vi "Convert Array to BMIH.vi"(1 "Array":u8[](array[numeric])) -> (0 "BITMAPINFOHEADER":T1)   [LabVIEW 2013, in "VRI.lvlib"]
uses:
  VRI.lvlib
  _Type Defs/BITMAPINFOHEADER.ctl
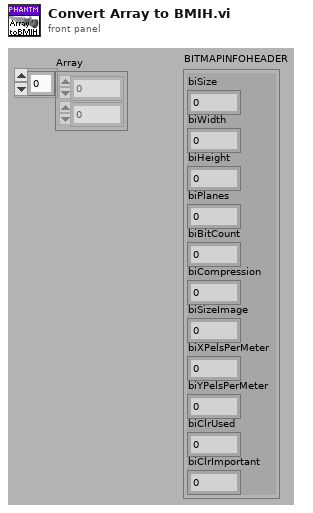
[diagram p1: front panel]
types:
  T1 = typedef "VRI.lvlib/BITMAPINFOHEADER.ctl" = cluster{"biSize":u32, "biWidth":i32, "biHeight":i32, "biPlanes":u16, "biBitCount":u16, "biCompression":u32, "biSizeImage":u32, "biXPelsPerMeter":i32, "biYPelsPerMeter":i32, "biClrUsed":u32, "biClrImportant":u32}
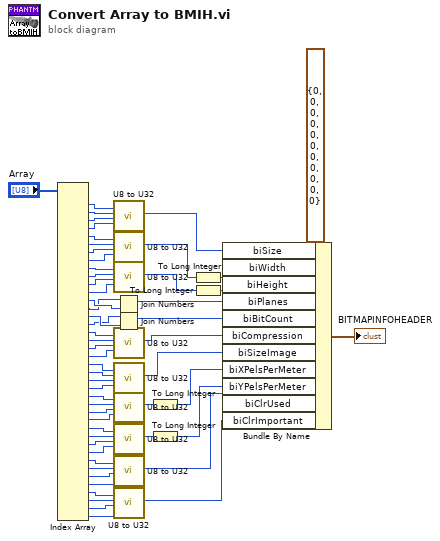
[diagram p0: block diagram]
diagram:
  n1 = Index Array(array="Array") -> (element #1=w7:u8, element #2=w4:u8, element #3=w6:u8, element #4=w5:u8, element #5=w9:u8, element #6=w10:u8, element #7=w11:u8, element #8=w12:u8, element #9=w13:u8, element #10=w14:u8, element #11=w15:u8, element #12=w16:u8, element #13=w56:u8, element #14=w55:u8, element #15=w58:u8, element #16=w57:u8, element #17=w23:u8, element #18=w24:u8, element #19=w25:u8, element #20=w26:u8, element #21=w27:u8, element #22=w28:u8, element #23=w29:u8, element #24=w30:u8, element #25=w35:u8, element #26=w36:u8, element #27=w37:u8, element #28=w38:u8, element #29=w39:u8, element #30=w40:u8, element #31=w41:u8, element #32=w42:u8, element #33=w44:u8, element #34=w45:u8, element #35=w46:u8, element #36=w47:u8, element #37=w48:u8, element #38=w49:u8, element #39=w50:u8, element #40=w51:u8)  [unwired: 40 in]
  n2 = call "U8 to U32.vi"("Byte1"=w7, "Byte2"=w4, "Byte3"=w6, "Byte4"=w5) -> ("U32"=w8:u32)  [unwired: 1 in, 14 out]
  n3 = call "U8 to U32.vi"("Byte1"=w9, "Byte2"=w10, "Byte3"=w11, "Byte4"=w12) -> ("U32"=w17:u32)  [unwired: 1 in, 14 out]
  n4 = call "U8 to U32.vi"("Byte1"=w13, "Byte2"=w14, "Byte3"=w15, "Byte4"=w16) -> ("U32"=w18:u32)  [unwired: 1 in, 14 out]
  n5 = Join Numbers(hi=w55, lo=w56) -> ((hi.lo)=w21:u16)
  n6 = Join Numbers(hi=w57, lo=w58) -> ((hi.lo)=w22:u16)
  n7 = call "U8 to U32.vi"("Byte1"=w23, "Byte2"=w24, "Byte3"=w25, "Byte4"=w26) -> ("U32"=w31:u32)  [unwired: 1 in, 14 out]
  n8 = call "U8 to U32.vi"("Byte1"=w27, "Byte2"=w28, "Byte3"=w29, "Byte4"=w30) -> ("U32"=w32:u32)  [unwired: 1 in, 14 out]
  n9 = call "U8 to U32.vi"("Byte1"=w35, "Byte2"=w36, "Byte3"=w37, "Byte4"=w38) -> ("U32"=w34:u32)  [unwired: 1 in, 14 out]
  n10 = call "U8 to U32.vi"("Byte1"=w39, "Byte2"=w40, "Byte3"=w41, "Byte4"=w42) -> ("U32"=w33:u32)  [unwired: 1 in, 14 out]
  n11 = call "U8 to U32.vi"("Byte1"=w44, "Byte2"=w45, "Byte3"=w46, "Byte4"=w47) -> ("U32"=w52:u32)  [unwired: 1 in, 14 out]
  n12 = call "U8 to U32.vi"("Byte1"=w48, "Byte2"=w49, "Byte3"=w50, "Byte4"=w51) -> ("U32"=w53:u32)  [unwired: 1 in, 14 out]
  n13 = To Long Integer(number=w34) -> (32bit integer=w54:i32)
  n14 = To Long Integer(number=w33) -> (32bit integer=w43:i32)
  n15 = To Long Integer(number=w17) -> (32bit integer=w19:i32)
  n16 = To Long Integer(number=w18) -> (32bit integer=w20:i32)
  n17 = Bundle By Name(cluster=T1 {"biSize"=0, "biWidth"=0, "biHeight"=0, "biPlanes"=0, "biBitCount"=0, "biCompression"=0, "biSizeImage"=0, "biXPelsPerMeter"=0, "biYPelsPerMeter"=0, "biClrUsed"=0, "biClrImportant"=0} ("BITMAPINFOHEADER"), "biSize"=w8, "biWidth"=w19, "biHeight"=w20, "biPlanes"=w21, "biBitCount"=w22, "biCompression"=w31, "biSizeImage"=w32, "biXPelsPerMeter"=w54, "biYPelsPerMeter"=w43, "biClrUsed"=w52, "biClrImportant"=w53) -> (→"BITMAPINFOHEADER":T1)
